vi "CRYUnflatten Hardware.vi"(11 "Unflatten Hardware#":string) -> (0 "Error?":bool=TRUE, 2 "Hardware":T1, 3 "Header info":T2={"Data type"="Data            ", "Version"=1, "Dimensions"=0})   [LabVIEW 2013]
uses:
  Typedef Control/CRY6175Hardware.ctl
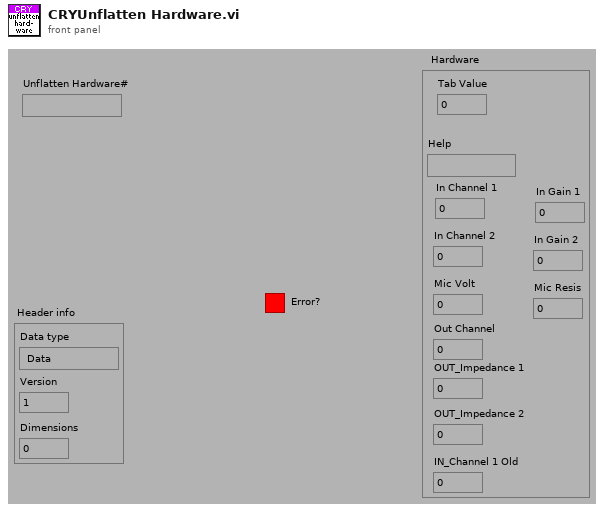
[diagram p1: front panel]
types:
  T1 = typedef "CRY6175Hardware.ctl" = cluster{"Tab Value":u16, "Help":string, "In Channel 1":u16, "In Channel 2":u16, "In Gain 1":i32, "In Gain 2":i32, "Mic Volt":i32, "Mic Resis":i32, "Out Channel":u16, "OUT_Impedance 1":u16, "OUT_Impedance 2":u16, "IN_Channel 1 Old":u16}
  T2 = cluster{"Data type":string, "Version":u16, "Dimensions":u8}
  T3 = cluster{"Tab Value":u16, "Help":string, "In Channel 1":u16, "In Channel 2":u16, "In Gain 1":i32, "In Gain 2":i32, "Mic Volt":i32, "Mic Resis":i32, "Out Channel":u16, "OUT_Impedance 1":u16, "OUT_Impedance 2":u16, "IN_Channel 1 Old":u16}
  T4 = cluster{"unsigned byte array[0]":u8, "unsigned byte array[1]":u8, "unsigned byte array[2]":u8}
  T5 = cluster{"Tab Value":u16, "Help":string, "In Channel 1":u16, "In Channel 2":u16, "In Gain 1":i32, "In Gain 2":i32, "Mic Volt":i32, "Mic Resis":i32, "Out Channel":u16, "OUT_Impedance 1":u16}
  T6 = cluster{"Tab Value":u16, "Help":string, "In Channel 1":u16, "In Channel 2":u16, "In Gain 1":i32, "In Gain 2":i32, "Mic Volt":i32, "Mic Resis":i32, "Out Channel":u16, "OUT_Impedance 1":u16, "OUT_Impedance 2":u16}
  T7 = cluster{"substring":string, u16, "unsigned byte array[2]":u8}
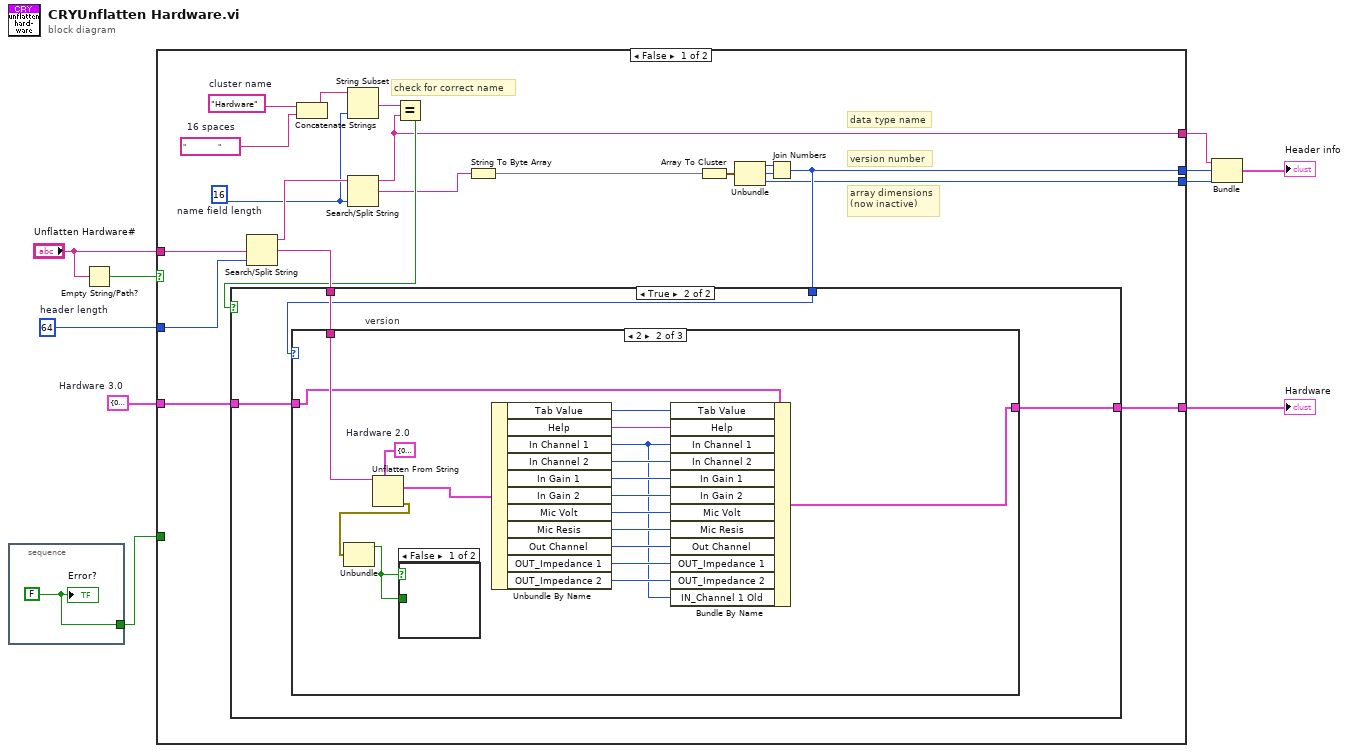
[diagram p0: block diagram]
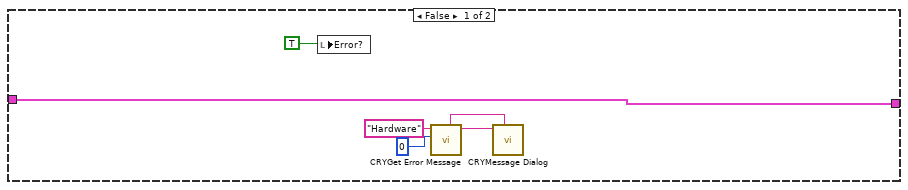
[diagram p2: hidden frame]
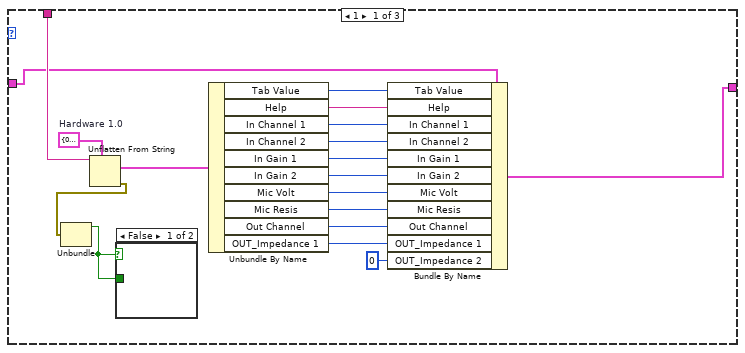
[diagram p3: hidden frame]
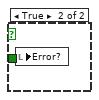
[diagram p4: hidden frame]
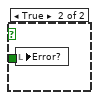
[diagram p5: hidden frame]
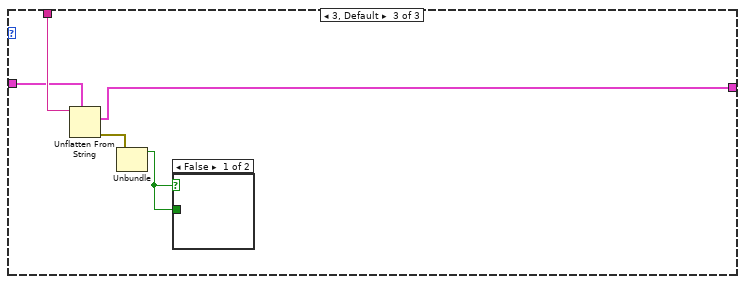
[diagram p6: hidden frame]
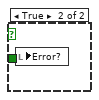
[diagram p7: hidden frame]
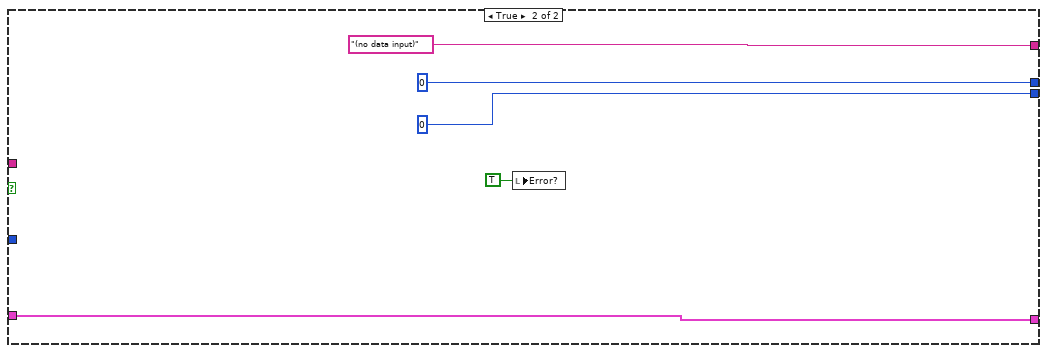
[diagram p8: hidden frame]
diagram:
  w2 = T3 {"Tab Value"=0, "Help"="", "In Channel 1"=0, "In Channel 2"=0, "In Gain 1"=0, "In Gain 2"=0, "Mic Volt"=0, "Mic Resis"=0, "Out Channel"=0, "OUT_Impedance 1"=0, "OUT_Impedance 2"=0, "IN_Channel 1 Old"=0}  # Hardware 3.0
  w7 = 64  # header length
  n1 = stacked-sequence {
    tunnel: [w11] -> w3
    frame #0 {
      w11 = FALSE
      "Error?" <- w11
    }
  }
  n2 = Empty String/Path?(string/path="Unflatten Hardware#") -> (empty?=w8:bool)
  n3 = case shown="False" w8 {
    tunnel: "Unflatten Hardware#" -> [w31 _]
    tunnel: w7 -> [w25 _]
    tunnel: [w22 u16 0] -> w5
    tunnel: [w14 u8 0] -> w6
    tunnel: [w15 "(no data input)" ("substring")] -> w4
    tunnel: w3 -> [_ _]
    tunnel: [w13 w86] -> w1
    tunnel: w2 -> [w12 w86]
    frame False {
      w19 = "                "  # 16 spaces
      w20 = "Hardware"  # cluster name
      w17 = 16  # name field length
      # "check for correct name"
      # "array dimensions\n(now inactive)"
      # "version number"
      # "data type name"
      n4 = Search/Split String(string=w31, offset (0)=w25) -> (substring before match=w24:string, match + rest of string=w26:string)  [unwired: 2 out]
      n5 = Concatenate Strings(w20, w19) -> (w18:string)
      n6 = String Subset(string=w18, length (rest)=w17) -> (substring=w16:string)  [unwired: 1 out]
      n7 = Search/Split String(string=w24, offset (0)=w17) -> (substring before match=w15:string, match + rest of string=w21:string)  [unwired: 2 out]
      n8 = Equal?(x=w16, y=w15) -> (x = y?=w23:bool)
      n9 = String To Byte Array(string=w21) -> (unsigned byte array=w30:u8[])
      n10 = Array To Cluster(array=w30) -> (cluster=w29:T4)
      n11 = Unbundle(w29) -> ("unsigned byte array[0]"=w28:u8, "unsigned byte array[1]"=w27:u8, "unsigned byte array[2]"=w14:u8)
      n12 = Join Numbers(hi=w28, lo=w27) -> ((hi.lo)=w22:u16)
      n13 = case shown="True" w23 {
        tunnel: w26 -> [_ w41]
        tunnel: w22 -> [_ w40]
        tunnel: [w36 w39] -> w13
        tunnel: w12 -> [w36 w38]
        frame False {
          n14 = local write "Error?"(TRUE) -> ()
          n15 = call "CRYGet Error Message.vi"("Error No"=0, "Kind"="Hardware") -> ("Message"=w33:string, "Window Title"=w32:string)  [unwired: 4 in, 4 out]
          n16 = call "CRYMessage Dialog.vi"("Window Title"=w32, "Message Content"=w33) -> ()  [unwired: 8 in, 2 out]
        }
        frame True {
          n17 = case "version" shown="2" w40 {
            tunnel: w41 -> [w59 w78 w84]
            tunnel: [w52 w72 w81] -> w39
            tunnel: w38 -> [w54 w74 w82]
            frame 1 {
              w56 = T5 {"Tab Value"=0, "Help"="", "In Channel 1"=0, "In Channel 2"=0, "In Gain 1"=0, "In Gain 2"=0, "Mic Volt"=0, "Mic Resis"=0, "Out Channel"=0, "OUT_Impedance 1"=0}  # Hardware 1.0
              n18 = Unflatten From String(type=w56, binary string=w59) -> (value=w55:T5, error out=w57:errorcluster)  [unwired: 1 in, 3 out]
              n19 = Unbundle(w57) -> ("status"=w58:bool)  [unwired: 2 out]
              n20 = case shown="False" w58 {
                tunnel: w58 -> [_ w60]
                frame False {
                }
                frame True {
                  n21 = local write "Error?"(w60) -> ()
                }
              }
              n22 = Unbundle By Name(w55) -> ("Tab Value"=w53:u16, "Help"=w51:string, "In Channel 1"=w50:u16, "In Channel 2"=w49:u16, "In Gain 1"=w48:i32, "In Gain 2"=w47:i32, "Mic Volt"=w46:i32, "Mic Resis"=w45:i32, "Out Channel"=w44:u16, "OUT_Impedance 1"=w43:u16)
              n23 = Bundle By Name(cluster=w54, "Tab Value"=w53, "Help"=w51, "In Channel 1"=w50, "In Channel 2"=w49, "In Gain 1"=w48, "In Gain 2"=w47, "Mic Volt"=w46, "Mic Resis"=w45, "Out Channel"=w44, "OUT_Impedance 1"=w43, "OUT_Impedance 2"=u16 0 ("OUT_Impedence 2")) -> (w52:T3)
            }
            frame 2 {
              w63 = T6 {"Tab Value"=0, "Help"="", "In Channel 1"=0, "In Channel 2"=0, "In Gain 1"=0, "In Gain 2"=0, "Mic Volt"=0, "Mic Resis"=0, "Out Channel"=0, "OUT_Impedance 1"=0, "OUT_Impedance 2"=0}  # Hardware 2.0
              n24 = Unflatten From String(type=w63, binary string=w78) -> (value=w75:T6, error out=w76:errorcluster)  [unwired: 1 in, 3 out]
              n25 = Unbundle(w76) -> ("status"=w77:bool)  [unwired: 2 out]
              n26 = case shown="False" w77 {
                tunnel: w77 -> [_ w79]
                frame False {
                }
                frame True {
                  n27 = local write "Error?"(w79) -> ()
                }
              }
              n28 = Unbundle By Name(w75) -> ("Tab Value"=w73:u16, "Help"=w71:string, "In Channel 1"=w61:u16, "In Channel 2"=w70:u16, "In Gain 1"=w69:i32, "In Gain 2"=w68:i32, "Mic Volt"=w67:i32, "Mic Resis"=w66:i32, "Out Channel"=w65:u16, "OUT_Impedance 1"=w64:u16, "OUT_Impedance 2"=w62:u16)
              n29 = Bundle By Name(cluster=w74, "Tab Value"=w73, "Help"=w71, "In Channel 1"=w61, "In Channel 2"=w70, "In Gain 1"=w69, "In Gain 2"=w68, "Mic Volt"=w67, "Mic Resis"=w66, "Out Channel"=w65, "OUT_Impedance 1"=w64, "OUT_Impedance 2"=w62, "IN_Channel 1 Old"=w61) -> (w72:T3)
            }
            frame 3, Default {
              n30 = Unflatten From String(type=w82, binary string=w84) -> (value=w81:T3, error out=w80:errorcluster)  [unwired: 1 in, 3 out]
              n31 = Unbundle(w80) -> ("status"=w83:bool)  [unwired: 2 out]
              n32 = case shown="False" w83 {
                tunnel: w83 -> [_ w85]
                frame False {
                }
                frame True {
                  n33 = local write "Error?"(w85) -> ()
                }
              }
            }
          }
        }
      }
    }
    frame True {
      n34 = local write "Error?"(TRUE ("Error?")) -> ()
    }
  }
  "Hardware" <- w1
  n35 = Bundle("substring"=w4, w5, "unsigned byte array[2]"=w6) -> (→"Header info":T7)  [unwired: 1 out]
